vi "Time-Y Circ Buffer.vi"(9 "buffer [1024]":i32=1024, 10 "Y in":dbl[](array[numeric]), 11 "XY in":cluster{timestamp[], dbl[]}[](array[cluster])) -> (3 "XY":cluster{timestamp[], dbl[]}[](array[cluster]))   [LabVIEW 2019, in "Instrument UI.Oxford1820.lvclass"]
uses:
  Instrument UI.Oxford1820.lvclass
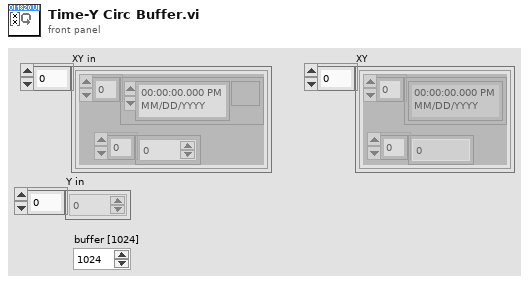
[diagram p1: front panel]
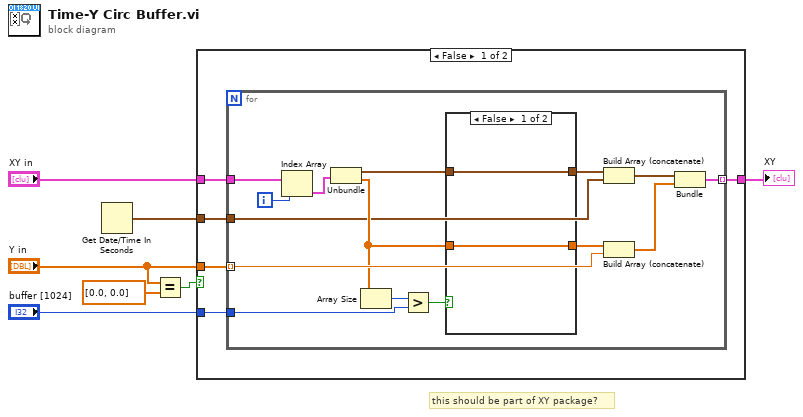
[diagram p0: block diagram]
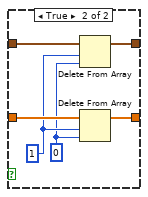
[diagram p2: hidden frame]
diagram:
  # "this should be part of XY package?"
  n1 = Get Date/Time In Seconds() -> (seconds since 1Jan1904=w4:timestamp)
  n2 = Equal?(x="Y in", y=dbl[] [0.0, 0.0]) -> (x = y?=w1:bool)
  n3 = case shown="False" w1 {
    tunnel: "buffer [1024]" -> [w12 _]
    tunnel: [w11 w36] -> w6
    tunnel: "XY in" -> [w10 w36]
    tunnel: w4 -> [w9 _]
    tunnel: "Y in" -> [w8 _]
    frame False {
      n4 = for {
        tunnel: w12 -> [w27]
        tunnel: w8 -> [w26] mode=indexing
        tunnel: [w25] -> w11 mode=indexing
        tunnel: w10 -> [w15]
        tunnel: w9 -> [w16]
        i -> [w13]
        n5 = Index Array(array=w15, index=w13) -> (element=w14:cluster{timestamp[], dbl[]})
        n6 = Unbundle(w14) -> (w19:timestamp[], w18:dbl[])
        n7 = Array Size(array=w18) -> (size(s)=w23:i32)
        n8 = Greater?(x=w23, y=w27) -> (0:w20:bool)
        n9 = case shown="False" w20 {
          tunnel: w18 -> [w29 w35]
          tunnel: [w29 w34] -> w22
          tunnel: w19 -> [w28 w32]
          tunnel: [w28 w31] -> w21
          frame False {
          }
          frame True {
            w30 = 0 ("length")
            w33 = 1 ("length")
            n10 = Delete From Array(array=w32, length=w33, index=w30) -> (array with subset deleted=w31:timestamp[])  [unwired: 1 out]
            n11 = Delete From Array(array=w35, length=w33, index=w30) -> (array with subset deleted=w34:dbl[])  [unwired: 1 out]
          }
        }
        n12 = Build Array (concatenate)(w21, w16) -> (w24:timestamp[])
        n13 = Build Array (concatenate)(w22, w26) -> (w17:dbl[])
        n14 = Bundle(w24, w17) -> (w25:cluster{timestamp[], dbl[]})  [unwired: 1 in]
      }
    }
    frame True {
    }
  }
  "XY" <- w6
